vi "Save 2D Array to Excel (SubVI).vi"(0 "File Path Input":path, 1 "Save (Enable/Signal)":bool, 2 "Save Interval (s)":dbl=1.0, 3 "Title Block Array":string[](array[string]), 4 "Column Header Array":string[](array[string]), 5 "Data Array (Table)":string[][](array[string]), 7 "File Configuration":T1={"Row Limit"=65500, "Default File Name"="Data", "New File Daily?"=TRUE, "Manual Save Interval?"=FALSE}, 9 "Change Save Location?":bool) -> (14 "File Path Output":path, 15 "Save Indicator":bool, 16 "# of Rows Saved":i32, 19 "Error Output":errorcluster)   [LabVIEW 2009]
panel:
  # "SAVE TO EXCEL SUBVI\nSave 2D Array (Table) to File"
  # "Created by Blake Otting 3/7/2007\nLast Updated 4/15/2010"
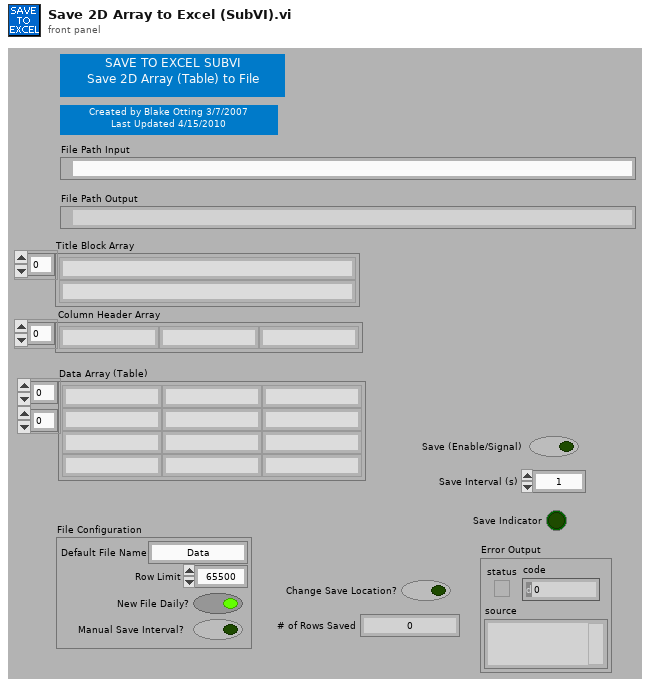
[diagram p1: front panel]
types:
  T1 = cluster{"Row Limit":i32, "Default File Name":string, "New File Daily?":bool, "Manual Save Interval?":bool}
  T2 = typedef "LVDateTimeRec.ctl" = cluster{"fractional second":dbl, "second":i32, "minute":i32, "hour":i32, "day of month":i32, "month":i32, "year":i32, "day of week":i32, "day of year":i32, "DST":i32}
  T3 = enum16{"open", "replace", "create", "open or create", "replace or create", "replace or create with confirmation"}
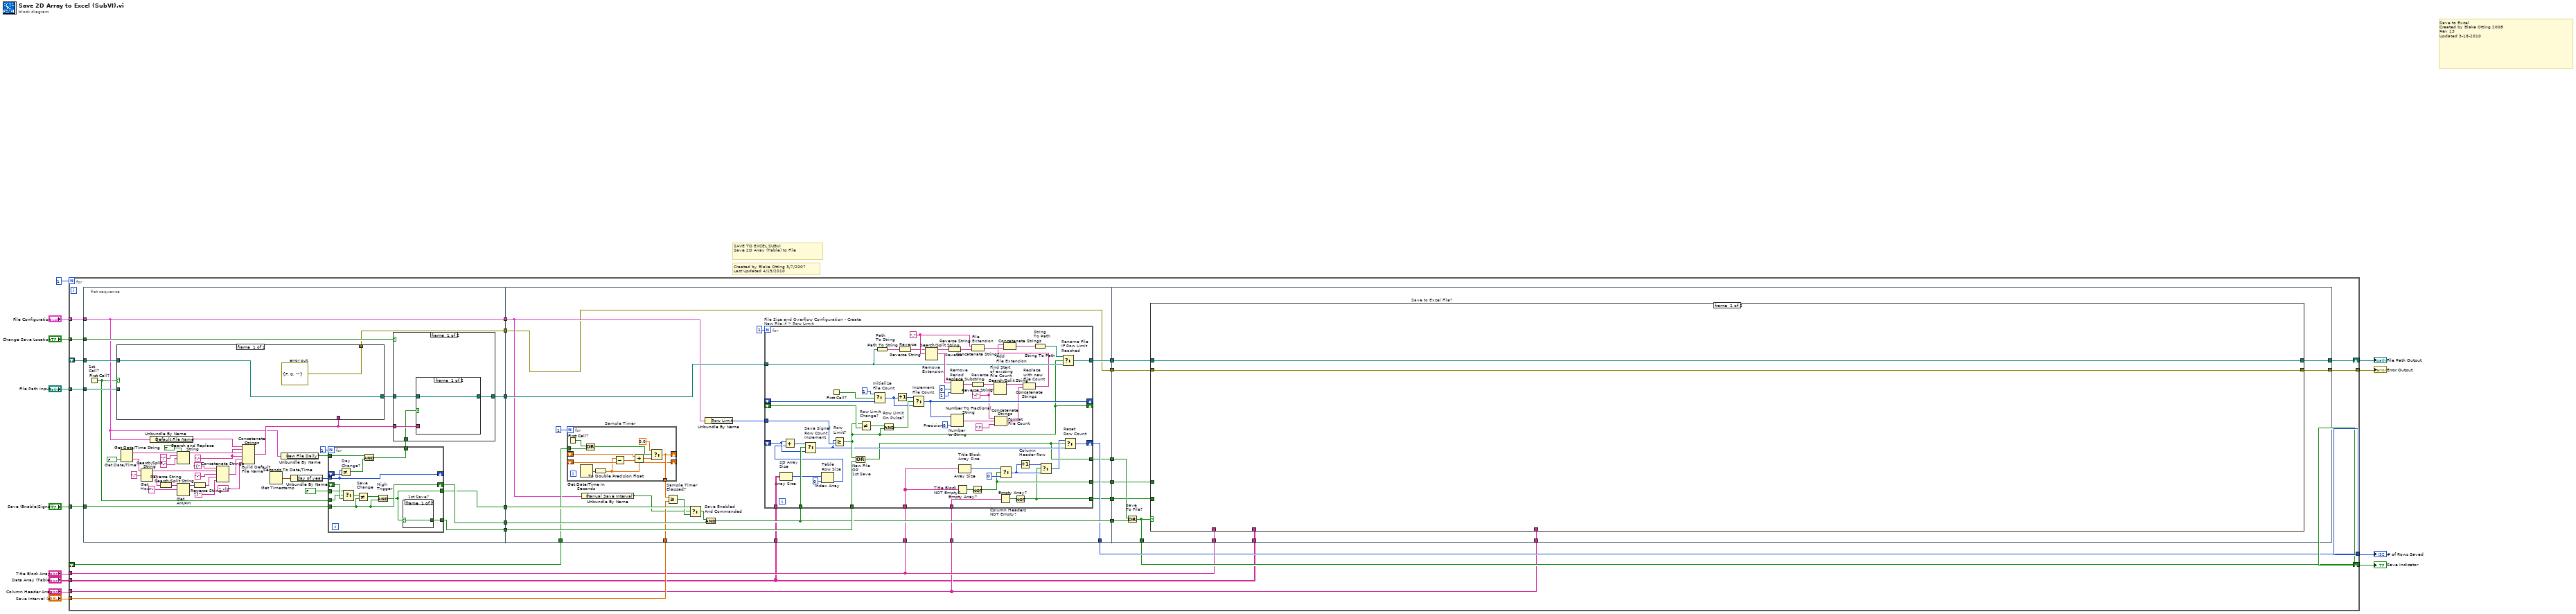
[diagram p0: block diagram]
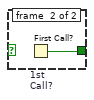
[diagram p2: hidden frame]
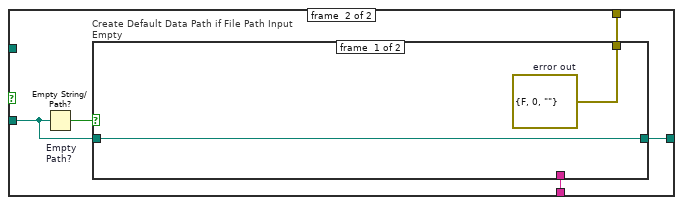
[diagram p3: hidden frame]
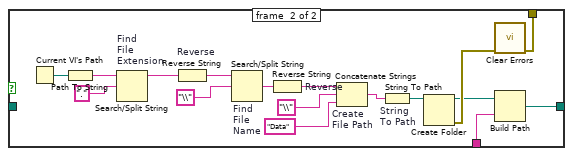
[diagram p4: hidden frame]
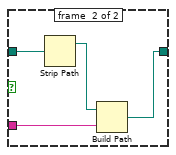
[diagram p5: hidden frame]
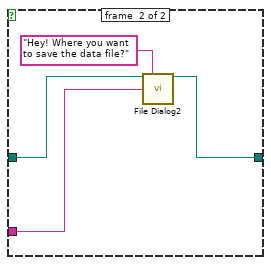
[diagram p6: hidden frame]
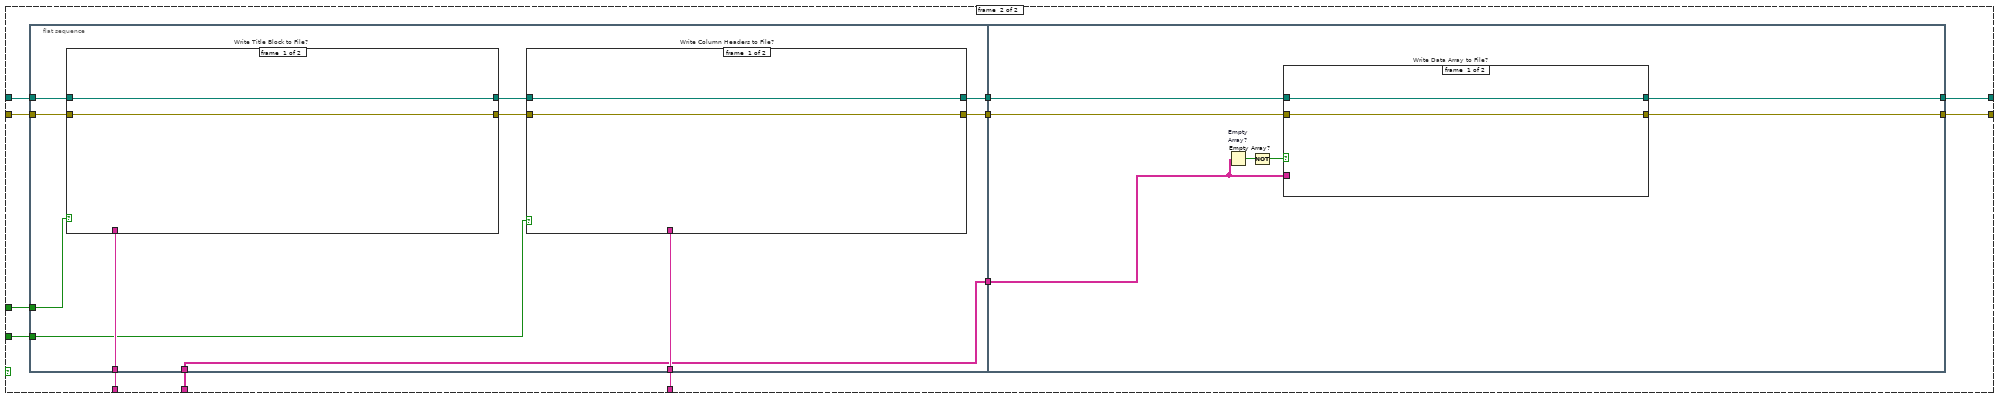
[diagram p7: hidden frame]
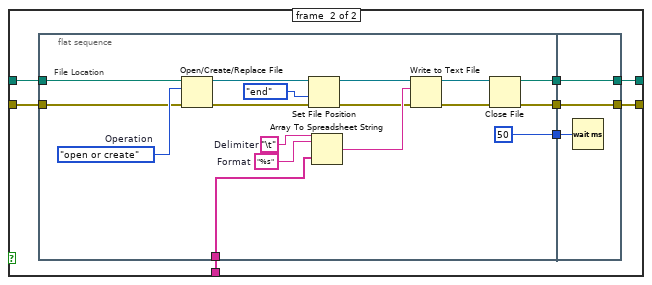
[diagram p8: hidden frame]
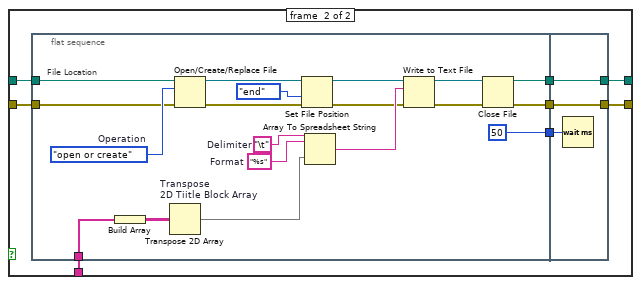
[diagram p9: hidden frame]
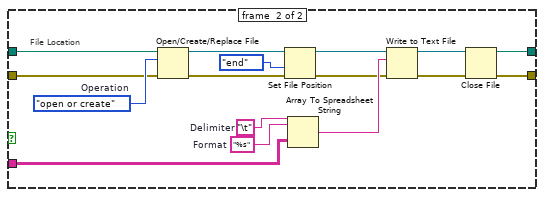
[diagram p10: hidden frame]
diagram:
  # "Created by Blake Otting 3/7/2007\nLast Updated 4/15/2010"
  # "SAVE TO EXCEL SUBVI\nSave 2D Array (Table) to File"
  # "Save to Excel\nCreated by Blake Otting 2008\nRev 13\nUpdated 3-18-2010"
  n1 = for {
    N: 1 -> [_]
    tunnel: "File Path Input" -> [w35]
    tunnel: "Change Save Location?" -> [w39]
    tunnel: "Save (Enable/Signal)" -> [w30]
    tunnel: "Data Array (Table)" -> [w18]
    tunnel: "Column Header Array" -> [w24]
    tunnel: "File Configuration" -> [w28]
    shift-right: [w32] -> w12
    shift-left: _ -> [w37]
    tunnel: "Save Interval (s)" -> [w31]
    tunnel: "Title Block Array" -> [w26]
    shift-right: [w17] -> w11
    shift-left: _ -> [w34]
    tunnel: [w33] -> w13
    tunnel: [w14] -> w1
    n2 = flat-sequence {
      tunnel: w34 -> [w50]
      tunnel: w35 -> [w49]
      tunnel: w39 -> [w43]
      tunnel: w28 -> [w42]
      tunnel: [w45] -> w38
      tunnel: w30 -> [w48]
      tunnel: [w47] -> w29
      tunnel: [w44] -> w27
      tunnel: [w42] -> w20
      tunnel: [w46] -> w19
      tunnel: [w40] -> w16
      tunnel: [w156] -> w36
      tunnel: w37 -> [w141]
      tunnel: w38 -> [w157]
      tunnel: [w150] -> w33
      tunnel: w31 -> [w139]
      tunnel: w29 -> [w154]
      tunnel: w27 -> [w151]
      tunnel: w26 -> [w149]
      tunnel: [w147] -> w25
      tunnel: w24 -> [w146]
      tunnel: [w145] -> w23
      tunnel: [w144] -> w22
      tunnel: [w138] -> w21
      tunnel: w20 -> [w137]
      tunnel: w19 -> [w148]
      tunnel: w18 -> [w135]
      tunnel: w16 -> [w134]
      tunnel: [w134] -> w15
      tunnel: w36 -> [w235]
      tunnel: w26 -> [w234]
      tunnel: w18 -> [w233]
      tunnel: w24 -> [w232]
      tunnel: [w231] -> w32
      tunnel: w25 -> [w227]
      tunnel: w23 -> [w230]
      tunnel: w22 -> [w229]
      tunnel: w21 -> [w228]
      tunnel: [w226] -> w17
      tunnel: w15 -> [w225]
      tunnel: [w224] -> w14
      frame #0 {
        w61 = "-" ("string")
        n3 = First Call? "1st\nCall?"() -> (First Call?: T/F=w41:bool)
        n4 = Get Date/Time String "Get Date/Time"(want seconds? (F)=FALSE) -> (date string=w56:string, time string=w55:string)  [unwired: 2 out]
        n5 = Search/Split String "Get\nHour"(string=w55, search string/char (-)=":" ("search string")) -> (substring before match=w66:string, match + rest of string=w63:string)  [unwired: 2 out]
        n6 = Unbundle By Name(w42) -> ("Default File Name"=w72:string)
        n7 = Reverse String(1:w63) -> (0:w64:string)
        n8 = Search and Replace String(replace all?=TRUE ("replace all? (F)"), input string=w56, search string="/", replace string="-" ("replace string (\"\")")) -> (result string=w71:string)  [unwired: 1 in, 6 out]
        n9 = Search/Split String "Get\nAM/PM"(string=w64, search string/char (-)=" ") -> (substring before match=w65:string)  [unwired: 3 out]
        n10 = Reverse String(1:w65) -> (0:w67:string)
        n11 = Concatenate Strings ("Build\nHour String")("{" ("string"), w66, "-" ("search string/char (-)"), w67, "}" ("string")) -> (w58:string)
        n12 = Concatenate Strings "Build Default\nFile Name"(w72, w61, w71, w61, w58, ".xls" ("string")) -> (w79:string)
        n13 = case shown="False" w41 {
          tunnel: w49 -> [_ w100]
          tunnel: [w96 w99] -> w51
          tunnel: w79 -> [_ w98]
          tunnel: w50 -> [w96 _]
          tunnel: [w95 w97] -> w40
          frame #0 {
            w95 = errorcluster {"status"=FALSE, "code"=0, "source"=""}  # error out
          }
          frame #1 {
            n14 = Empty String/Path? "Empty\nPath?"(string/path=w100) -> (empty?=w101:bool)
            n15 = case "Create Default Data Path if File Path Input Empty" shown="False" w101 {
              tunnel: [w103 w106] -> w99
              tunnel: w100 -> [w103 _]
              tunnel: w98 -> [_ w105]
              tunnel: [w102 w104] -> w97
              frame #0 {
                w102 = errorcluster {"status"=FALSE, "code"=0, "source"=""}  # error out
              }
              frame #1 {
                n16 = Current VI's Path() -> (path=w112:path)
                n17 = Path To String(path=w112) -> (string=w118:string)
                n18 = Search/Split String "Find\nFile \nExtension"(string=w118, search string/char (-)=".") -> (substring before match=w117:string)  [unwired: 1 in, 2 out]
                n19 = Reverse String "Reverse"(1:w117) -> (0:w116:string)
                n20 = Search/Split String "Find\nFile \nName"(string=w116, search string/char (-)="\\") -> (match + rest of string=w114:string)  [unwired: 1 in, 2 out]
                n21 = Reverse String "Reverse"(1:w114) -> (0:w113:string)
                n22 = Concatenate Strings "Create\nFile Path"(w113, "\\", "Data") -> (w120:string)
                n23 = String To Path "String\nTo Path"(string=w120) -> (path=w110:path)
                n24 = Create Folder(path (use dialog)=w110) -> (created path=w107:path, error out=w109:errorcluster)  [unwired: 2 in, 1 out]
                n25 = call <vilib>:"Clear Errors.vi"("error in (no error)"=w109) -> ("error out"=w104:errorcluster)  [unwired: 6 in]
                n26 = Build Path(base path=w107, name or relative path=w105) -> (appended path=w106:path)
              }
            }
          }
        }
        n27 = Seconds To Date/Time "Get Timestamp"() -> (date time rec=w77:T2)  [unwired: 2 out]
        n28 = Unbundle By Name(w42) -> ("New File Daily?"=w73:bool)
        n29 = Unbundle By Name(w77) -> ("day of year"=w74:i32)
        n30 = for {
          N: 1 -> [_]
          tunnel: w48 -> [w91]
          shift-right: [w91] -> w47
          shift-left: _ -> [w85]
          tunnel: w74 -> [w89]
          shift-right: [w89] -> _
          shift-left: _ -> [w90]
          tunnel: w73 -> [w87]
          tunnel: [w86] -> w76
          tunnel: [w83] -> w45
          tunnel: [w82] -> w44
          tunnel: w41 -> [w81]
          tunnel: FALSE -> [w80]
          n31 = Not Equal? "Day\nChange?"(x=w89, y=w90) -> (x != y?=w88:bool)
          n32 = Select(t=w80, s=w81, f=w85) -> (s? t:f=w84:bool)
          n33 = Not Equal? "Save\nChange"(x=w84, y=w91) -> (x != y?=w92:bool)
          n34 = And(x=w87, y=w88) -> (x .and. y?=w86:bool)
          n35 = And "High\nTrigger"(x=w92, y=w91) -> (x .and. y?=w82:bool)
          n36 = case "1st Save?" shown="True" w82 {
            selector: w82 -> [w93 _]
            tunnel: [w93 w94] -> w83
            frame #0 {
            }
            frame #1 {
              n37 = First Call? "1st\nCall?"() -> (First Call?: T/F=w94:bool)
            }
          }
        }
        n38 = case shown="False" w43 {
          tunnel: w51 -> [w124 w133]
          tunnel: w79 -> [w123 w131]
          tunnel: w76 -> [w122 _]
          tunnel: [w121 w130] -> w46
          frame #0 {
            n39 = case shown="True" w122 {
              tunnel: w124 -> [w125 w129]
              tunnel: w123 -> [_ w127]
              tunnel: [w125 w126] -> w121
              frame #0 {
              }
              frame #1 {
                n40 = Strip Path(path=w129) -> (stripped path=w128:path)  [unwired: 1 out]
                n41 = Build Path(base path=w128, name or relative path=w127) -> (appended path=w126:path)
              }
            }
          }
          frame #1 {
            n42 = call "File Dialog2"("start path"=w133, "prompt"="Hey! Where you want to save the data file?", "default name"=w131) -> ("selected path"=w130:path)  [unwired: 4 in, 8 out]
          }
        }
      }
      frame #1 {
        n43 = for "Sample Timer" {
          N: 1 -> [_]
          shift-right: [w165] -> _
          shift-left: _ -> [w168]
          shift-right: [w159] -> _
          shift-left: _ -> [w167]
          tunnel: [w165] -> w142
          tunnel: w141 -> [w161]
          n44 = First Call?() -> (First Call?: T/F=w160:bool)
          n45 = Get Date/Time In Seconds() -> (seconds since 1Jan1904=w166:timestamp)
          n46 = Or(x=w160, y=w161) -> (x .or. y?=w162:bool)
          n47 = To Double Precision Float(number=w166) -> (double precision float=w159:dbl)
          n48 = Subtract(x=w159, y=w167) -> (x-y=w158:dbl)
          n49 = Add(x=w168, y=w158) -> (x+y=w164:dbl)
          n50 = Select(t=0.0, s=w162, f=w164) -> (s? t:f=w165:dbl)
        }
        n51 = Unbundle By Name(w137) -> ("Manual Save Interval?"=w136:bool)
        n52 = Greater Or Equal? "Sample Timer\nElapsed?"(x=w142, y=w139) -> (x >= y?=w140:bool)
        n53 = Select(t=w151, s=w136, f=w140) -> (s? t:f=w155:bool)
        n54 = And "Save Enabled\nAnd Commanded"(x=w155, y=w154) -> (x .and. y?=w156:bool)
        n55 = Unbundle By Name(w137) -> ("Row Limit"=w153:i32)
        n56 = for "File Size and Overflow Configuration - Create New File if > Row Limit" {
          N: 1 -> [_]
          tunnel: w157 -> [w223]
          tunnel: w156 -> [w222]
          shift-right: [w220] -> w150
          shift-left: _ -> [w171]
          tunnel: w153 -> [w221]
          shift-right: [w188] -> _
          shift-left: _ -> [w219]
          tunnel: w149 -> [w184]
          shift-right: [w213] -> _
          shift-left: _ -> [w191]
          tunnel: w148 -> [w202]
          tunnel: [w194] -> w147
          tunnel: w146 -> [w186]
          tunnel: [w178] -> w144
          tunnel: [w177] -> w138
          tunnel: [w175] -> w145
          tunnel: w135 -> [w174]
          w211 = "." ("search string/char (-)")
          w195 = "-("
          w217 = i16 0  # Precision
          n57 = Array Size "2D Array\nSize"(array=w174) -> (size(s)=w173:i32[])
          n58 = Index Array "Table\nRow Size"(array=w173, index=0) -> (element=w170:i32)
          n59 = Add(x=w171, y=w170) -> (x+y=w169:i32)
          n60 = Select "Save Signal\nRow Count\nIncrement"(t=w169, s=w222, f=w171) -> (s? t:f=w176:i32)
          n61 = First Call?() -> (First Call?: T/F=w192:bool)
          n62 = Greater Or Equal? "Row\nLimit?"(x=w176, y=w221) -> (x >= y?=w188:bool)
          n63 = Or "New File\nOR\n1st Save"(x=w188, y=w223) -> (x .or. y?=w175:bool)
          n64 = Not Equal? "Row Limit\nChange?"(x=w188, y=w219) -> (x != y?=w214:bool)
          n65 = Select "Initialize\nFile Count"(t=i16 1, s=w192, f=w191) -> (s? t:f=w190:i16)
          n66 = Path To String "Path\nTo String"(path=w202) -> (string=w204:string)
          n67 = And "Row Limit\nOn Pulse?"(x=w214, y=w188) -> (x .and. y?=w218:bool)
          n68 = Increment(x=w190) -> (x+1=w215:i16)
          n69 = Reverse String "Reverse"(1:w204) -> (0:w205:string)
          n70 = Select "Increment\nFile Count"(t=w215, s=w218, f=w190) -> (s? t:f=w213:i16)
          n71 = Search/Split String "Remove\nExtension"(string=w205, search string/char (-)=w211) -> (substring before match=w206:string, match + rest of string=w207:string)  [unwired: 2 out]
          n72 = Reverse String "Reverse"(1:w206) -> (0:w203:string)
          n73 = Replace Substring "Remove\nPeriod"(2:1 ("length (len. of substring)"), 3:0 ("offset (0)"), 5:w207) -> (1:w208:string)  [unwired: 2 out]
          n74 = Number To Fractional String "Number\nto String"(number=w213, precision (6)=w217) -> (F-format string=w216:string)  [unwired: 2 in]
          n75 = Empty Array? "Title Block\nNOT Empty?"(array=w184) -> (empty?=w185:bool)
          n76 = Array Size "Title Block\nArray Size"(array=w184) -> (size(s)=w183:i32)
          n77 = Reverse String "Reverse"(1:w208) -> (0:w200:string)
          n78 = Not(x=w185) -> (.not. x?=w178:bool)
          n79 = Concatenate Strings "File\nExtension"(w211, w203) -> (w197:string)
          n80 = Search/Split String "Find Start\nof existing\nFile Count"(string=w200, search string/char (-)=w195) -> (substring before match=w199:string)  [unwired: 1 in, 2 out]
          n81 = Concatenate Strings "Format\nFile Count"(w195, w216, ")") -> (w198:string)
          n82 = Empty Array? "Column Headers\nNOT Empty?"(array=w186) -> (empty?=w187:bool)
          n83 = Select(t=w183, s=w178, f=0 ("t")) -> (s? t:f=w181:i32)
          n84 = Not(x=w187) -> (.not. x?=w177:bool)
          n85 = Increment "Column\nHeader Row"(x=w181) -> (x+1=w180:i32)
          n86 = Concatenate Strings "Replace\nwith new\nFile Count"(w199, w198) -> (w189:string)
          n87 = Concatenate Strings "Add\nFile Extension"(w189, w197) -> (w196:string)
          n88 = String To Path "String\nTo Path"(string=w196) -> (path=w212:path)
          n89 = Select(t=w180, s=w177, f=w181) -> (s? t:f=w179:i32)
          n90 = Select "Rename File\nIF Row Limit\nReached"(t=w212, s=w188, f=w202) -> (s? t:f=w194:path)
          n91 = Select "Reset\nRow Count"(t=w179, s=w175, f=w176) -> (s? t:f=w220:i32)
        }
      }
      frame #2 {
        n92 = Or "Save\nTo File?"(x=w230, y=w235) -> (x .or. y?=w231:bool)
        n93 = case "Save to Excel File?" shown="True" w231 {
          tunnel: w234 -> [_ w247]
          tunnel: w233 -> [_ w249]
          tunnel: w232 -> [_ w248]
          tunnel: w229 -> [_ w246]
          tunnel: w228 -> [_ w245]
          tunnel: w227 -> [w237 w243]
          tunnel: [w237 w239] -> w226
          tunnel: w225 -> [w236 w242]
          tunnel: [w236 w238] -> w224
          frame #0 {
          }
          frame #1 {
            n94 = flat-sequence {
              tunnel: w247 -> [w260]
              tunnel: w248 -> [w259]
              tunnel: w249 -> [w256]
              tunnel: [w256] -> w244
              tunnel: w246 -> [w258]
              tunnel: w245 -> [w257]
              tunnel: w243 -> [w255]
              tunnel: w242 -> [w254]
              tunnel: [w252] -> w241
              tunnel: [w250] -> w240
              tunnel: w244 -> [w328]
              tunnel: w241 -> [w325]
              tunnel: w240 -> [w326]
              tunnel: [w324] -> w239
              tunnel: [w323] -> w238
              frame #0 {
                n95 = case "Write Title Block to File?" shown="False" w258 {
                  tunnel: w260 -> [_ w300]
                  tunnel: w255 -> [w291 w298]
                  tunnel: w254 -> [w292 w297]
                  tunnel: [w292 w295] -> w253
                  tunnel: [w291 w293] -> w251
                  frame #0 {
                  }
                  frame #1 {
                    n96 = flat-sequence "Write to Excel File" {
                      tunnel: w300 -> [w306]
                      tunnel: [u32 50 ("milliseconds to wait")] -> w299
                      tunnel: w298 -> [w304]
                      tunnel: w297 -> [w303]
                      tunnel: [w302] -> w296
                      tunnel: [w301] -> w294
                      tunnel: w299 -> [w322]
                      tunnel: [w321] -> w295
                      tunnel: w296 -> [w321]
                      tunnel: [w320] -> w293
                      tunnel: w294 -> [w320]
                      frame #0 {
                        w316 = "\t"  # Delimiter
                        w315 = "%s"  # Format
                        w318 = T3."open or create"  # Operation
                        # "File Location"
                        n97 = Build Array(w306) -> (w308:string[][])
                        n98 = Transpose 2D Array "Transpose\n2D Tiitle Block Array"(2D array=w308) -> (transposed array=w307:string[][])
                        n99 = Open/Create/Replace File(file path (use dialog)=w304, error in=w303, operation (0:open)=w318) -> (refnum out=w309:refnum<file>, error out=w310:errorcluster)  [unwired: 3 in, 1 out]
                        n100 = Set File Position(refnum=w309, from (0:start)=enum16{"start", "end", "current"}."end", error in=w310) -> (refnum out=w311:refnum<file>, error out=w312:errorcluster)  [unwired: 1 in]
                        n101 = Array To Spreadsheet String(delimiter (Tab)=w316, array=w307, 3:w315) -> (spreadsheet string=w317:string)
                        n102 = Write to Text File(file (use dialog)=w311, text=w317, error in=w312) -> (refnum out=w313:refnum<file>, error out=w314:errorcluster)  [unwired: 1 in, 1 out]
                        n103 = Close File(refnum=w313, error in=w314) -> (path=w301:path, error out=w302:errorcluster)
                      }
                      frame #1 {
                        n104 = Wait (ms)(milliseconds to wait=w322) -> ()  [unwired: 1 out]
                      }
                    }
                  }
                }
                n105 = case "Write Column Headers to File?" shown="False" w257 {
                  tunnel: w259 -> [_ w270]
                  tunnel: w253 -> [w262 w268]
                  tunnel: [w262 w263] -> w252
                  tunnel: w251 -> [w261 w266]
                  tunnel: [w261 w265] -> w250
                  frame #0 {
                  }
                  frame #1 {
                    n106 = flat-sequence "Write to Excel File" {
                      tunnel: w270 -> [w275]
                      tunnel: [u32 50 ("milliseconds to wait")] -> w269
                      tunnel: w268 -> [w274]
                      tunnel: [w273] -> w267
                      tunnel: w266 -> [w272]
                      tunnel: [w271] -> w264
                      tunnel: w269 -> [w290]
                      tunnel: [w289] -> w263
                      tunnel: w267 -> [w289]
                      tunnel: [w288] -> w265
                      tunnel: w264 -> [w288]
                      frame #0 {
                        w284 = "\t"  # Delimiter
                        w283 = "%s"  # Format
                        w286 = T3."open or create"  # Operation
                        # "File Location"
                        n107 = Open/Create/Replace File(file path (use dialog)=w272, error in=w274, operation (0:open)=w286) -> (refnum out=w277:refnum<file>, error out=w278:errorcluster)  [unwired: 3 in, 1 out]
                        n108 = Set File Position(refnum=w277, from (0:start)=enum16{"start", "end", "current"}."end", error in=w278) -> (refnum out=w279:refnum<file>, error out=w280:errorcluster)  [unwired: 1 in]
                        n109 = Array To Spreadsheet String(delimiter (Tab)=w284, array=w275, 3:w283) -> (spreadsheet string=w285:string)
                        n110 = Write to Text File(file (use dialog)=w279, text=w285, error in=w280) -> (refnum out=w281:refnum<file>, error out=w282:errorcluster)  [unwired: 1 in, 1 out]
                        n111 = Close File(refnum=w281, error in=w282) -> (path=w271:path, error out=w273:errorcluster)
                      }
                      frame #1 {
                        n112 = Wait (ms)(milliseconds to wait=w290) -> ()  [unwired: 1 out]
                      }
                    }
                  }
                }
              }
              frame #1 {
                n113 = Empty Array? "Empty\nArray?"(array=w328) -> (empty?=w329:bool)
                n114 = Not(x=w329) -> (.not. x?=w327:bool)
                n115 = case "Write Data Array to File?" shown="True" w327 {
                  tunnel: w328 -> [_ w336]
                  tunnel: w326 -> [w331 w335]
                  tunnel: w325 -> [w330 w334]
                  tunnel: [w331 w332] -> w324
                  tunnel: [w330 w333] -> w323
                  frame #0 {
                  }
                  frame #1 {
                    w344 = "\t"  # Delimiter
                    w343 = "%s"  # Format
                    w346 = T3."open or create"  # Operation
                    # "File Location"
                    n116 = Open/Create/Replace File(file path (use dialog)=w335, error in=w334, operation (0:open)=w346) -> (refnum out=w337:refnum<file>, error out=w338:errorcluster)  [unwired: 3 in, 1 out]
                    n117 = Set File Position(refnum=w337, from (0:start)=enum16{"start", "end", "current"}."end", error in=w338) -> (refnum out=w339:refnum<file>, error out=w340:errorcluster)  [unwired: 1 in]
                    n118 = Array To Spreadsheet String(delimiter (Tab)=w344, array=w336, 3:w343) -> (spreadsheet string=w345:string)
                    n119 = Write to Text File(file (use dialog)=w339, text=w345, error in=w340) -> (refnum out=w341:refnum<file>, error out=w342:errorcluster)  [unwired: 1 in, 1 out]
                    n120 = Close File(refnum=w341, error in=w342) -> (path=w332:path, error out=w333:errorcluster)
                  }
                }
              }
            }
          }
        }
      }
    }
  }
  "# of Rows Saved" <- w13
  "Save Indicator" <- w12
  "File Path Output" <- w11
  "Error Output" <- w1
